vi "GCD of P(x) and Q(x) (DBL).vi"(8 "algorithm":u16(ring) items=["Euclidean", "Approximate GCD"], 9 "tolerance":dbl=1e-08 format="%#.6g", 10 "Q(x)":dbl[](array[numeric]), 11 "P(x)":dbl[](array[numeric])) -> (0 "error":i32, 3 "Greatest Common Divisor":dbl[](array[numeric]))   [LabVIEW 2024, in "NI_AALPro.lvlib"]
doc: "<p>Computes the greatest common divisor for two polynomials <strong>P(x)</strong> and <strong>Q(x)</strong> with the <strong>tolerance</strong> you specify. The data types you wire to the <strong>P(x)</strong> and <strong>Q(x)</strong> inputs determine the polymorphic instance to use.</p>"
uses:
  NI_AALPro.lvlib
  RMS (DBL).vi
  Polynomial GCD Pair (DBL).vi
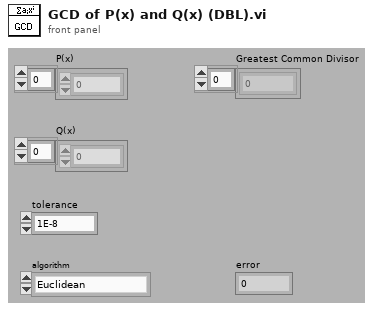
[diagram p1: front panel]
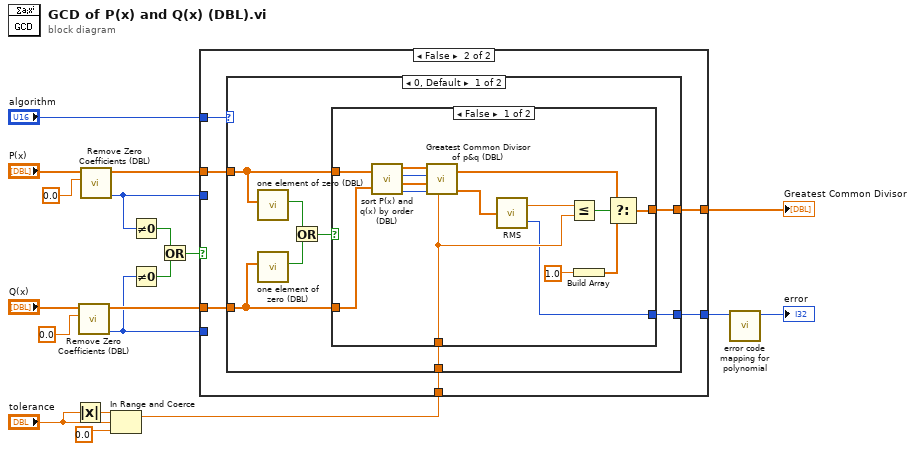
[diagram p0: block diagram]
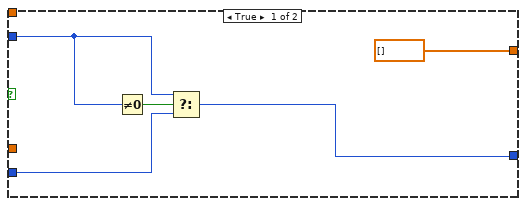
[diagram p2: hidden frame]
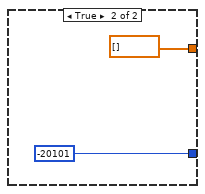
[diagram p3: hidden frame]
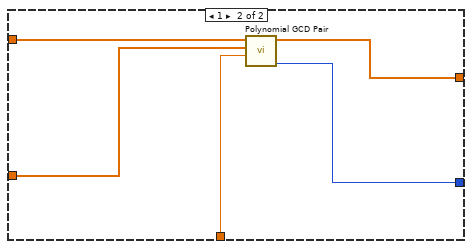
[diagram p4: hidden frame]
diagram:
  n1 = Absolute Value(x="tolerance") -> (abs(x)=w10:dbl)
  n2 = call "Remove Zero Coefficients (DBL).vi"("threshold"=0.0, "P(x) In"="Q(x)") -> ("error"=w5:i32, "P(x) Out"=w15:dbl[])  [unwired: 7 in, 1 out]
  n3 = call "Remove Zero Coefficients (DBL).vi"("threshold"=0.0, "P(x) In"="P(x)") -> ("error"=w6:i32, "P(x) Out"=w16:dbl[])  [unwired: 7 in, 1 out]
  n4 = In Range and Coerce(upper limit=w10, x="tolerance", lower limit=0.0) -> (coerced(x)=w9:dbl)  [unwired: 1 out]
  n5 = Not Equal To 0?(x=w6) -> (x != 0?=w4:bool)
  n6 = Not Equal To 0?(x=w5) -> (x != 0?=w3:bool)
  n7 = Or(x=w4, y=w3) -> (x .or. y?=w2:bool)
  n8 = case shown="False" w2 {
    tunnel: [dbl[] [] ("BDL") w30] -> w19
    tunnel: w16 -> [_ w29]
    tunnel: w15 -> [_ w28]
    tunnel: [w20 w27] -> w8
    tunnel: w9 -> [_ w26]
    tunnel: w6 -> [w22 _]
    tunnel: w5 -> [w21 _]
    tunnel: "algorithm" -> [_ w25]
    frame True {
      n9 = Not Equal To 0?(x=w22) -> (x != 0?=w23:bool)
      n10 = Select(t=w22, s=w23, f=w21) -> (s? t:f=w20:i32)
    }
    frame False {
      n11 = case shown="0, Default" w25 {
        tunnel: [w38 w57] -> w30
        tunnel: w29 -> [w35 w60]
        tunnel: w28 -> [w33 w59]
        tunnel: [w32 w56] -> w27
        tunnel: w26 -> [w31 w58]
        frame 0, Default {
          n12 = call "one element of zero (DBL).vi"("Array in"=w35) -> ("equal [0]?"=w36:bool)  [unwired: 10 in]
          n13 = call "one element of zero (DBL).vi"("Array in"=w33) -> ("equal [0]?"=w34:bool)  [unwired: 10 in]
          n14 = Or(x=w36, y=w34) -> (x .or. y?=w37:bool)
          n15 = case shown="False" w37 {
            tunnel: w35 -> [w53 _]
            tunnel: w33 -> [w52 _]
            tunnel: [w51 dbl[] []] -> w38
            tunnel: [w39 -20101 ("coef. of poly are all zero")] -> w32
            tunnel: w31 -> [w40 _]
            frame False {
              n16 = call "sort P(x) and q(x) by order (DBL).vi"("p"=w53, "q"=w52) -> ("high order polynomial"=w50:dbl[], "high order"=w49:i32, "low order polynomial"=w48:dbl[], "low order"=w47:i32)
              n17 = call "Greatest Common Divisor of p&q (DBL).vi"("p"=w50, "order of p"=w49, "q"=w48, "order of q"=w47, "threshold"=w40) -> ("greatest common factor"=w46:dbl[], "rest"=w42:dbl[])
              n18 = call-poly "RMS.vi"("X"=w42) -> ("rms value"=w41:dbl, "error"=w39:i32)
              n19 = Less Or Equal?(x=w41, y=w40) -> (x <= y?=w43:bool)
              n20 = Build Array(1.0) -> (w44:dbl[])
              n21 = Select(t=w46, s=w43, f=w44) -> (s? t:f=w51:dbl[])
            }
            frame True {
            }
          }
        }
        frame 1 {
          n22 = call-poly "Polynomial GCD Pair.vi"("tolerance"=w58, "Q(x)"=w59, "P(x)"=w60) -> ("error"=w56:i32, "Greatest Common Divisor"=w57:dbl[])  [unwired: 5 in, 2 out]
        }
      }
    }
  }
  "Greatest Common Divisor" <- w19
  n23 = call "error code mapping for polynomial.vi"("error in"=w8) -> ("error out"=→"error":i32)  [unwired: 10 in]
